vi "Neue Log Datei anlegen.vi"(8 "error in (no error)":errorcluster caption="Fehler (Eingang, kein Fehler)") -> (0 "error out":errorcluster caption="Fehler (Ausgang)")   [LabVIEW 2015, in "Schedule Modul.lvlib"]
uses:
  Schedule Modul.lvlib
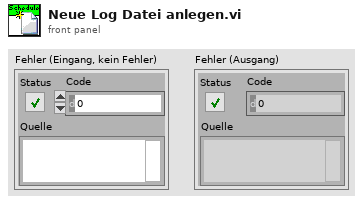
[diagram p1: front panel]
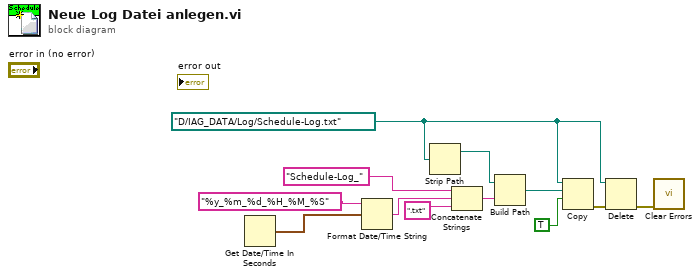
[diagram p0: block diagram]
diagram:
  w8 = path "D:/IAG_DATA/Log/Schedule-Log.txt" ("Datei")
  n1 = Get Date/Time In Seconds() -> (seconds since 1Jan1904=w10:timestamp)
  n2 = Format Date/Time String(time format string (%c)="%y_%m_%d_%H_%M_%S" ("Zeitformatierungs-String (%c)"), seconds (now)=w10) -> (date/time string=w11:string)  [unwired: 1 in]
  n3 = Strip Path(path=w8) -> (stripped path=w7:path)  [unwired: 1 out]
  n4 = Concatenate Strings("Schedule-Log_" ("name or relative path"), w11, ".txt" ("string")) -> (w4:string)
  n5 = Build Path(base path=w7, name or relative path=w4) -> (appended path=w3:path)
  n6 = Copy(9:TRUE ("overwrite (F)"), 10:w3, 11:w8) -> (0:w1:errorcluster)  [unwired: 2 in, 2 out]
  n7 = Delete(path (use dialog)=w8, error in=w1) -> (error out=w12:errorcluster)  [unwired: 3 in, 2 out]
  n8 = call <vilib>:"Clear Errors.vi"("error in (no error)"=w12) -> ()  [unwired: 5 in, 2 out]
